vi "heart.vi"() -> ()   [LabVIEW 2013]
uses:
  <vilib>/Instr/_visa.llb/VISA Configure Serial Port (Instr).vi
  <vilib>/Utility/file.llb/Write To Spreadsheet File (DBL).vi
panel:
  out "BMP":string
  in  "exit":bool
  in  "Start":bool
  out "Grafik P-Q-R-S-T":dbl(graph)
  in  "pause":bool
  in  "Baud Rate":u32=9600
  in  "Port Serial":refnum<visa-resource-name>
  # "CONTROL BLOCK"
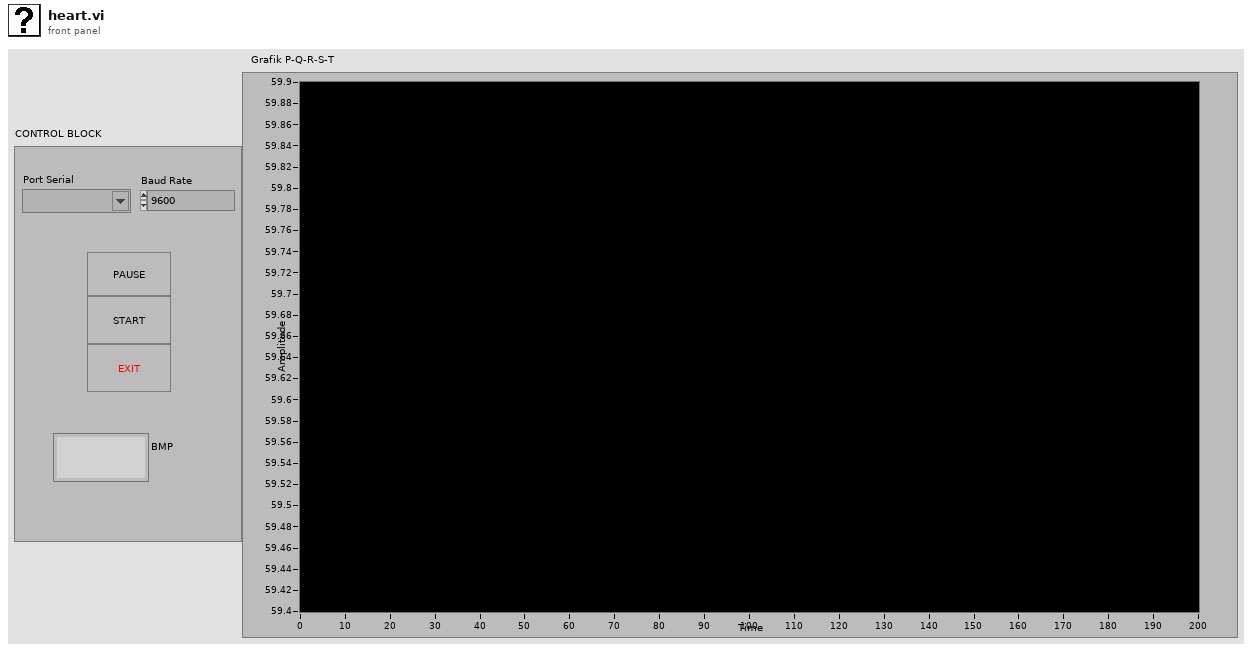
[diagram p1: front panel]
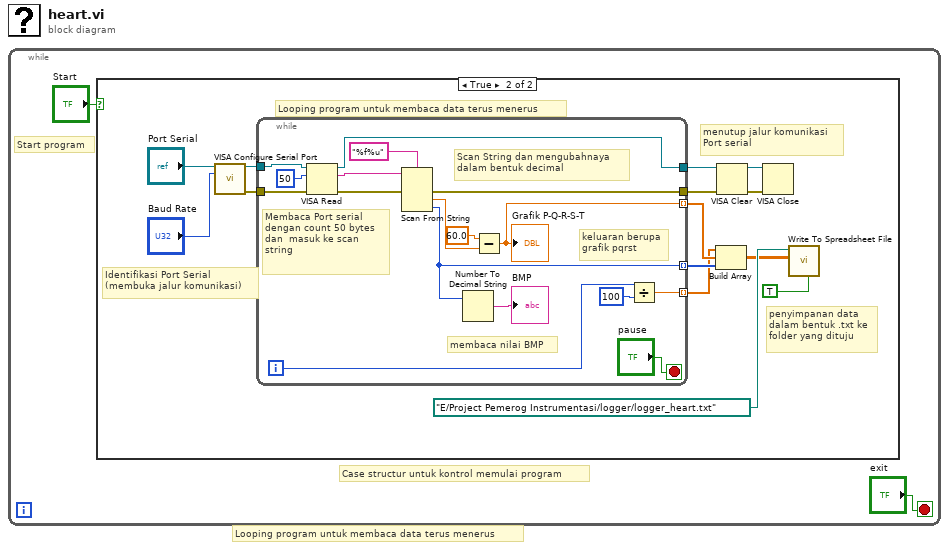
[diagram p0: block diagram]
diagram:
  # "Looping program untuk membaca data terus menerus"
  n1 = while {
    stop <- "exit" stop-if-true
    # "Case structur untuk kontrol memulai program"
    # "Start program"
    n2 = case shown="True" "Start" {
      frame False {
      }
      frame True {
        # "Looping program untuk membaca data terus menerus"
        # "menutup jalur komunikasi\nPort serial"
        # "penyimpanan data\ndalam bentuk .txt ke\nfolder yang dituju"
        # "Identifikasi Port Serial\n(membuka jalur komunikasi)"
        n3 = call-poly "VISA Configure Serial Port"("VISA resource name"="Port Serial", "baud rate (9600)"="Baud Rate") -> ("VISA resource name out"=w14:refnum<visa-resource-name>, "error out"=w13:errorcluster)  [unwired: 12 in]
        n4 = while {
          tunnel: w14 -> [w33]
          tunnel: w13 -> [w32]
          tunnel: [w27] -> w12
          tunnel: [w24] -> w9
          tunnel: [w21] -> w5 mode=indexing
          tunnel: [w17] -> w4 mode=indexing
          tunnel: [w18] -> w3 mode=indexing
          i -> [w20]
          stop <- "pause" stop-if-true
          # "membaca nilai BMP"
          # "keluaran berupa\ngrafik pqrst"
          # "Scan String dan mengubahnaya \ndalam bentuk decimal"
          # "Membaca Port serial\ndengan count 50 bytes\ndan  masuk ke scan string"
          n5 = VISA Read(VISA resource name=w33, byte count=u32 50, error in (no error)=w32) -> (VISA resource name out=w27:refnum<visa-resource-name>, read buffer=w29:string, error out=w30:errorcluster)  [unwired: 1 out]
          n6 = Scan From String(format string="%f%u", input string=w29, error in=w30) -> (error out=w24:errorcluster, output 1=w26:dbl, output 2=w21:u32)  [unwired: 3 in, 2 out]
          n7 = Number To Decimal String(number=w21) -> (decimal integer string=→"BMP":string)  [unwired: 1 in]
          n8 = Subtract(x=60.0, y=w26) -> (x-y=w17:dbl)
          "Grafik P-Q-R-S-T" <- w17
          n9 = Divide(x=w20, y=100) -> (x/y=w18:dbl)
        }
        n10 = Build Array(w3, w4, w5) -> (w7:dbl[][])
        n11 = VISA Clear(VISA resource name=w12, error in (no error)=w9) -> (VISA resource name out=w11:refnum<visa-resource-name>, error out=w10:errorcluster)
        n12 = VISA Close(VISA resource name=w11, error in (no error)=w10) -> ()  [unwired: 1 out]
        n13 = call-poly <vilib>:"Write To Spreadsheet File.vi"("transpose? (no:F)"=TRUE, "2D data"=w7, "file path (dialog if empty)"=path "E:/Project Pemerog Instrumentasi/logger/logger_heart.txt") -> ()  [unwired: 5 in, 1 out]
      }
    }
  }
